vi "GetModeSatus.vi"(7 "Tab Control":refnum<vi>, 8 "error in (no error)":errorcluster {"code" format="%.0x"}, 11 "instrument handle":refnum<k15>) -> (0 "error out":errorcluster {"code" format="%.0x"}, 1 "number":u32, 2 "appended array":bool[](array[boolean]), 3 "instrument handle out":refnum<k15>)   [LabVIEW 2015, in "MyToolsFunction.lvlib"]
uses:
  ICcamera/MyToolsFunction.lvlib
  Tek shared libraries/SerialCommunication.lvlib
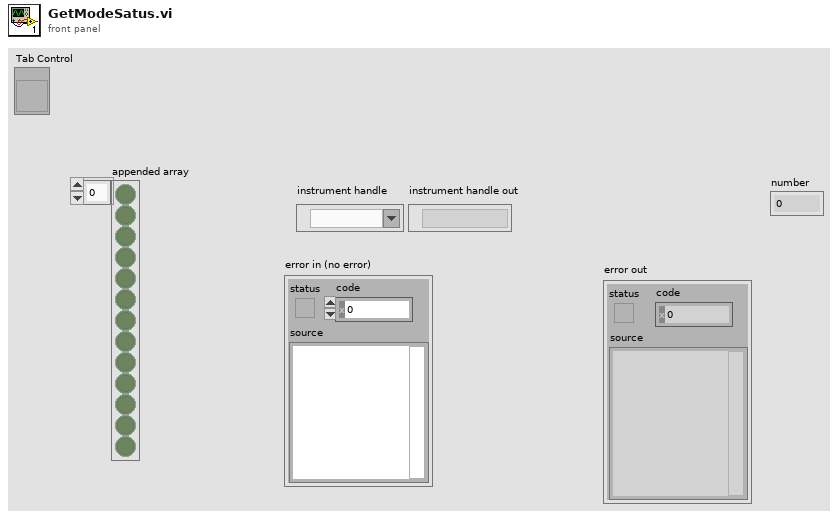
[diagram p1: front panel]
types:
  T1 = enum32{"CW", "AM", "FM", "PM", "FSK", "Sweep", "Burst"}
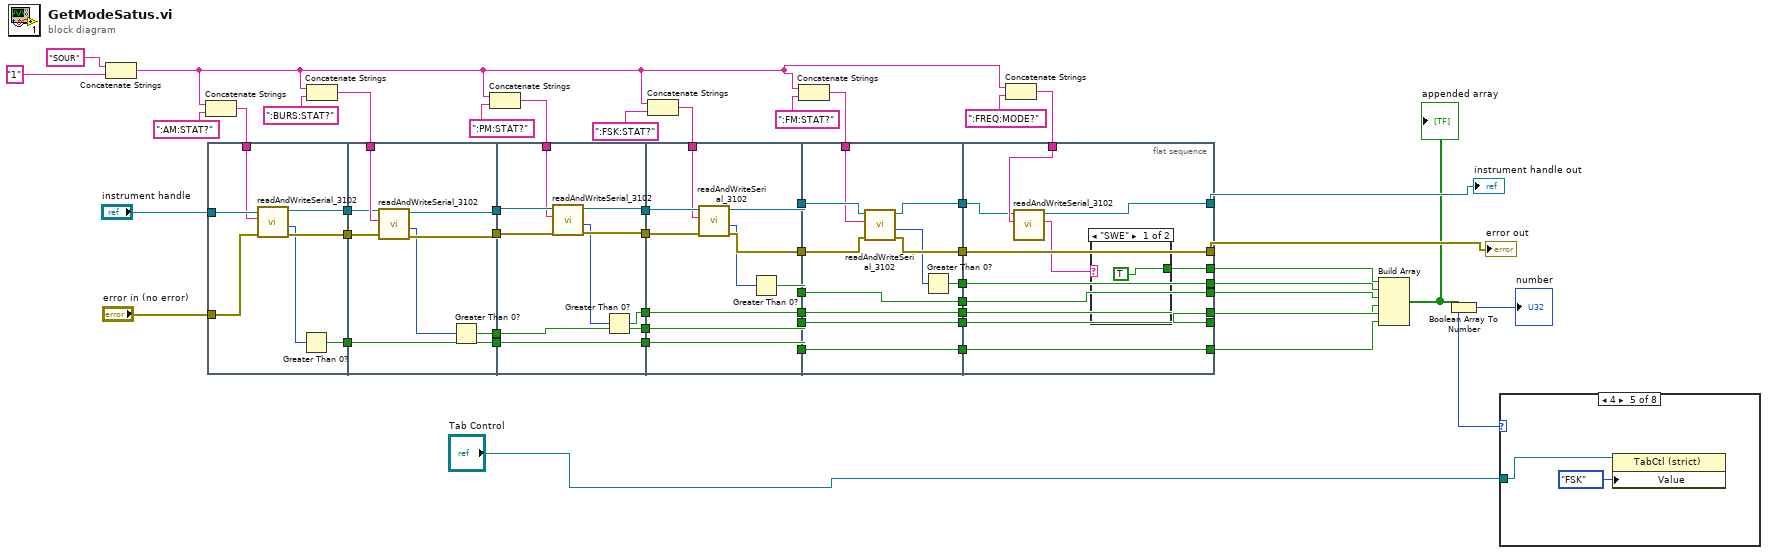
[diagram p0: block diagram]
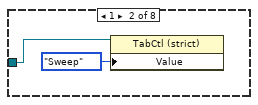
[diagram p3: hidden frame]
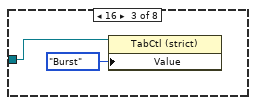
[diagram p4: hidden frame]
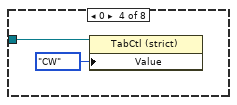
[diagram p5: hidden frame]
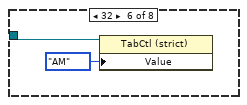
[diagram p6: hidden frame]
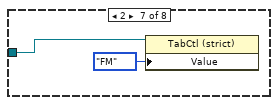
[diagram p7: hidden frame]
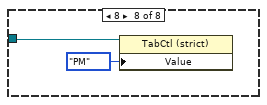
[diagram p8: hidden frame]
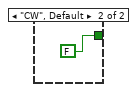
[diagram p9: hidden frame]
diagram:
  n1 = Concatenate Strings("SOUR" ("Write Buffer (\"\")"), "1" ("Write Buffer (\"\")")) -> (w4:string)
  n2 = Concatenate Strings(w4, ":AM:STAT?" ("Write Buffer (\"\")")) -> (w34:string)
  n3 = flat-sequence {
    tunnel: "instrument handle" -> [w60]
    tunnel: "error in (no error)" -> [w56]
    tunnel: w34 -> [w59]
    tunnel: [w58] -> w49
    tunnel: [w57] -> w48
    tunnel: [w55] -> w30
    tunnel: w49 -> [w65]
    tunnel: w48 -> [w68]
    tunnel: w45 -> [w66]
    tunnel: [w67] -> w44
    tunnel: [w64] -> w35
    tunnel: [w63] -> w31
    tunnel: w30 -> [w63]
    tunnel: [w61] -> w26
    tunnel: w44 -> [w77]
    tunnel: w42 -> [w73]
    tunnel: [w76] -> w38
    tunnel: [w74] -> w36
    tunnel: w35 -> [w75]
    tunnel: [w72] -> w32
    tunnel: w31 -> [w72]
    tunnel: [w71] -> w27
    tunnel: w26 -> [w71]
    tunnel: [w69] -> w24
    tunnel: w40 -> [w83]
    tunnel: w38 -> [w87]
    tunnel: w36 -> [w84]
    tunnel: w32 -> [w82]
    tunnel: w27 -> [w81]
    tunnel: w24 -> [w78]
    tunnel: [w86] -> w21
    tunnel: [w85] -> w20
    tunnel: [w82] -> w19
    tunnel: [w81] -> w18
    tunnel: [w79] -> w17
    tunnel: [w78] -> w16
    tunnel: w21 -> [w91]
    tunnel: w20 -> [w94]
    tunnel: w19 -> [w98]
    tunnel: w18 -> [w97]
    tunnel: w17 -> [w96]
    tunnel: w16 -> [w95]
    tunnel: w14 -> [w92]
    tunnel: [w90] -> w12
    tunnel: [w93] -> w11
    tunnel: [w98] -> w10
    tunnel: [w97] -> w9
    tunnel: [w96] -> w8
    tunnel: [w95] -> w7
    tunnel: [w88] -> w6
    tunnel: [w104] -> w13
    tunnel: [w105] -> w23
    tunnel: [w106] -> w25
    tunnel: [w107] -> w28
    tunnel: [w108] -> w33
    tunnel: [w101] -> w37
    tunnel: [w109] -> w39
    tunnel: w12 -> [w109]
    tunnel: w11 -> [w102]
    tunnel: w10 -> [w108]
    tunnel: w9 -> [w107]
    tunnel: w8 -> [w106]
    tunnel: w7 -> [w105]
    tunnel: w6 -> [w104]
    tunnel: w3 -> [w103]
    tunnel: [w99] -> w2
    frame #0 {
      n4 = call "readAndWriteSerial_3102.vi"("error in (no error)"=w56, "Write Buffer (\"\")"=w59, "instrument handle"=w60) -> ("error out"=w57:errorcluster, "converted number"=w54:i32, "instrument handle out"=w58:refnum<k15>)  [unwired: 5 in, 1 out]
      n5 = Greater Than 0?(x=w54) -> (x > 0?=w55:bool)
    }
    frame #1 {
      n6 = call "readAndWriteSerial_3102.vi"("error in (no error)"=w68, "Write Buffer (\"\")"=w66, "instrument handle"=w65) -> ("error out"=w67:errorcluster, "converted number"=w62:i32, "instrument handle out"=w64:refnum<k15>)  [unwired: 5 in, 1 out]
      n7 = Greater Than 0?(x=w62) -> (x > 0?=w61:bool)
    }
    frame #2 {
      n8 = call "readAndWriteSerial_3102.vi"("error in (no error)"=w77, "Write Buffer (\"\")"=w73, "instrument handle"=w75) -> ("error out"=w76:errorcluster, "converted number"=w70:i32, "instrument handle out"=w74:refnum<k15>)  [unwired: 5 in, 1 out]
      n9 = Greater Than 0?(x=w70) -> (x > 0?=w69:bool)
    }
    frame #3 {
      n10 = call "readAndWriteSerial_3102.vi"("error in (no error)"=w87, "Write Buffer (\"\")"=w83, "instrument handle"=w84) -> ("error out"=w86:errorcluster, "converted number"=w80:i32, "instrument handle out"=w85:refnum<k15>)  [unwired: 5 in, 1 out]
      n11 = Greater Than 0?(x=w80) -> (x > 0?=w79:bool)
    }
    frame #4 {
      n12 = call "readAndWriteSerial_3102.vi"("error in (no error)"=w91, "Write Buffer (\"\")"=w92, "instrument handle"=w94) -> ("error out"=w90:errorcluster, "converted number"=w89:i32, "instrument handle out"=w93:refnum<k15>)  [unwired: 5 in, 1 out]
      n13 = Greater Than 0?(x=w89) -> (x > 0?=w88:bool)
    }
    frame #5 {
      n14 = call "readAndWriteSerial_3102.vi"("Write Buffer (\"\")"=w103, "instrument handle"=w102) -> ("Read Buffer"=w100:string, "instrument handle out"=w101:refnum<k15>)  [unwired: 6 in, 2 out]
      n15 = case shown="\"SWE\"" w100 {
        tunnel: [TRUE FALSE] -> w99
        frame "SWE" {
        }
        frame "CW", Default {
        }
      }
    }
  }
  n16 = Concatenate Strings(w4, ":BURS:STAT?" ("Write Buffer (\"\")")) -> (w45:string)
  n17 = Concatenate Strings(w4, ":PM:STAT?" ("Write Buffer (\"\")")) -> (w42:string)
  n18 = Concatenate Strings(w4, ":FSK:STAT?" ("Write Buffer (\"\")")) -> (w40:string)
  n19 = Concatenate Strings(w4, ":FM:STAT?" ("Write Buffer (\"\")")) -> (w14:string)
  n20 = Concatenate Strings(w4, ":FREQ:MODE?" ("Write Buffer (\"\")")) -> (w3:string)
  n21 = Build Array(w2, w13, w25, w23, w28, w33) -> (w29:bool[])
  "appended array" <- w29
  n22 = Boolean Array To Number(Boolean array=w29) -> (number=w22:u32)
  "number" <- w22
  n23 = case shown="4" w22 {
    tunnel: "Tab Control" -> [_ w113 w115 w117 w118 w121 w123 w125]
    frame Default {
    }
    frame 1 {
      n24 = property class="TabCtl (strict)"(reference=w113, "Value"=T1."Sweep") -> ()  [unwired: 1 in, 2 out]
    }
    frame 16 {
      n25 = property class="TabCtl (strict)"(reference=w115, "Value"=T1."Burst") -> ()  [unwired: 1 in, 2 out]
    }
    frame 0 {
      n26 = property class="TabCtl (strict)"(reference=w117, "Value"=T1."CW") -> ()  [unwired: 1 in, 2 out]
    }
    frame 4 {
      n27 = property class="TabCtl (strict)"(reference=w118, "Value"=T1."FSK") -> ()  [unwired: 1 in, 2 out]
    }
    frame 32 {
      n28 = property class="TabCtl (strict)"(reference=w121, "Value"=T1."AM") -> ()  [unwired: 1 in, 2 out]
    }
    frame 2 {
      n29 = property class="TabCtl (strict)"(reference=w123, "Value"=T1."FM") -> ()  [unwired: 1 in, 2 out]
    }
    frame 8 {
      n30 = property class="TabCtl (strict)"(reference=w125, "Value"=T1."PM") -> ()  [unwired: 1 in, 2 out]
    }
  }
  "instrument handle out" <- w37
  "error out" <- w39
